vi "UTILITY Search Pattern 1D Array.vi"(10 "Search Item":string, 11 "1D Array":string[](array[string])) -> (3 "Index":i32)   [LabVIEW 2016]
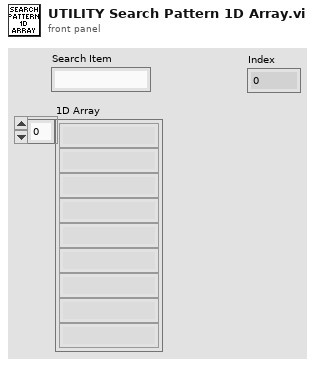
[diagram p1: front panel]
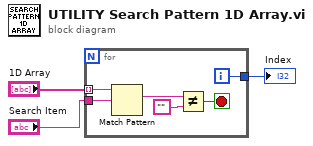
[diagram p0: block diagram]
diagram:
  n1 = for {
    tunnel: "1D Array" -> [w9] mode=indexing
    tunnel: [w8] -> w1
    tunnel: "Search Item" -> [w6]
    i -> [w8]
    stop <- w5 stop-if-true
    n2 = Match Pattern(string=w9, regular expression=w6) -> (match substring=w4:string)  [unwired: 1 in, 3 out]
    n3 = Not Equal?(x=w4, y="") -> (x != y?=w5:bool)
  }
  "Index" <- w1
